vi "Digitizer Fetch and Analyze.vi"(3 "Offset":dbl, 4 "Published Data Id":string[](array[string]), 5 "Vertical Coupling":i32(ring)=1 items=["AC", "DC", "Ground"], 6 "Vertical Range (V)":dbl=2.0 format="%_3g", 7 "Pins":string[](array[string])=["Xout"], 8 "error in (no error)":errorcluster, 9 "Min Record Length":i32=1000 caption="Record Length", 10 "Min. Sample Rate":dbl=1000000.0 caption="Sample Rate" format="%#_6p", 11 "Semiconductor Module Context":T1) -> (0 "error out":errorcluster)   [LabVIEW 2014]
doc: "Example: Measurement Library\n\nRecommended Input Signal: 100 kHz, 2 Vpp, sine wave\n\nDevices Supported: Refer to NI Example Finders\n\nLabVIEW Description:\n\nThis example illustrates fetching scalar measurements from NI-SCOPE, such as period and rise time calculations. \n\nSome common horizontal and vertical parameters are configured for the oscilloscope. The property node is used to set the reference level units, and the low, middle and high reference levels. For more information about measurement library parameters, see the NI-SCOPE VI Reference Help file. \n\nAfter the Read VI is called to acquire a waveform, the Fetch Measurement Stats VI is used to perform the desired scalar measurement analysis on the waveform. NI-SCOPE keeps a history of each measurement's results, which allows it to retrieve the statistics computed over multiple acquisitions. These statistics include the mean, standard deviation, min, max and number of acquisitions used in the statistics. The statistics are updated once per acquisition when the measurement is fetched. The Clear Stats VI clears this history."
uses:
  <vilib>/NI_TestStand_SemiconductorModule/NI_TestStand_Semiconductor_Module.lvlibp/PinMap/General/SemiconductorModuleContext.ctl
  <vilib>/NI_TestStand_SemiconductorModule/NI_TestStand_Semiconductor_Module.lvlibp/PinMap/Advanced/Custom Instruments/GetSessionDataSinglePinSingleInstr.vi
  <instrlib>/niScope/Configure/Trigger/niScope Configure Trigger Immediate.vi
  <instrlib>/niScope/Acquire/niScope Read WDT.vi
  <vilib>/measure/matone.llb/Extract Single Tone Information 1 Chan.vi
  <vilib>/NI_TestStand_SemiconductorModule/NI_TestStand_Semiconductor_Module.lvlibp/PinMap/General/Publish/PublishDataDoubleFunctionalTest.vi
  <vilib>/NI_TestStand_SemiconductorModule/NI_TestStand_Semiconductor_Module.lvlibp
  <vilib>/measure/NI_MAPro.lvlib
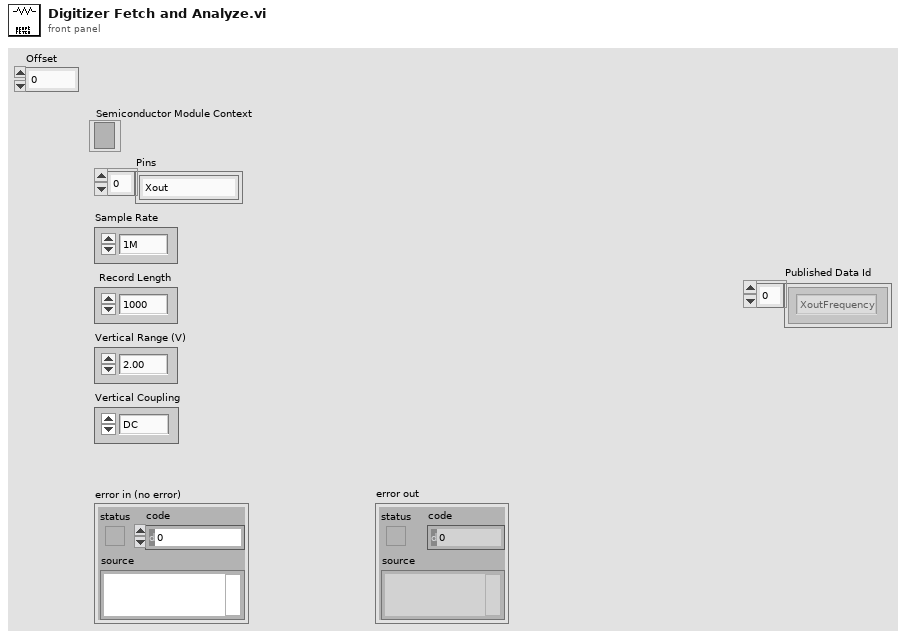
[diagram p1: front panel]
types:
  T1 = typedef "NI_TestStand_Semiconductor_Module.lvlibp/SemiconductorModuleContext.ctl" = refnum<k7>
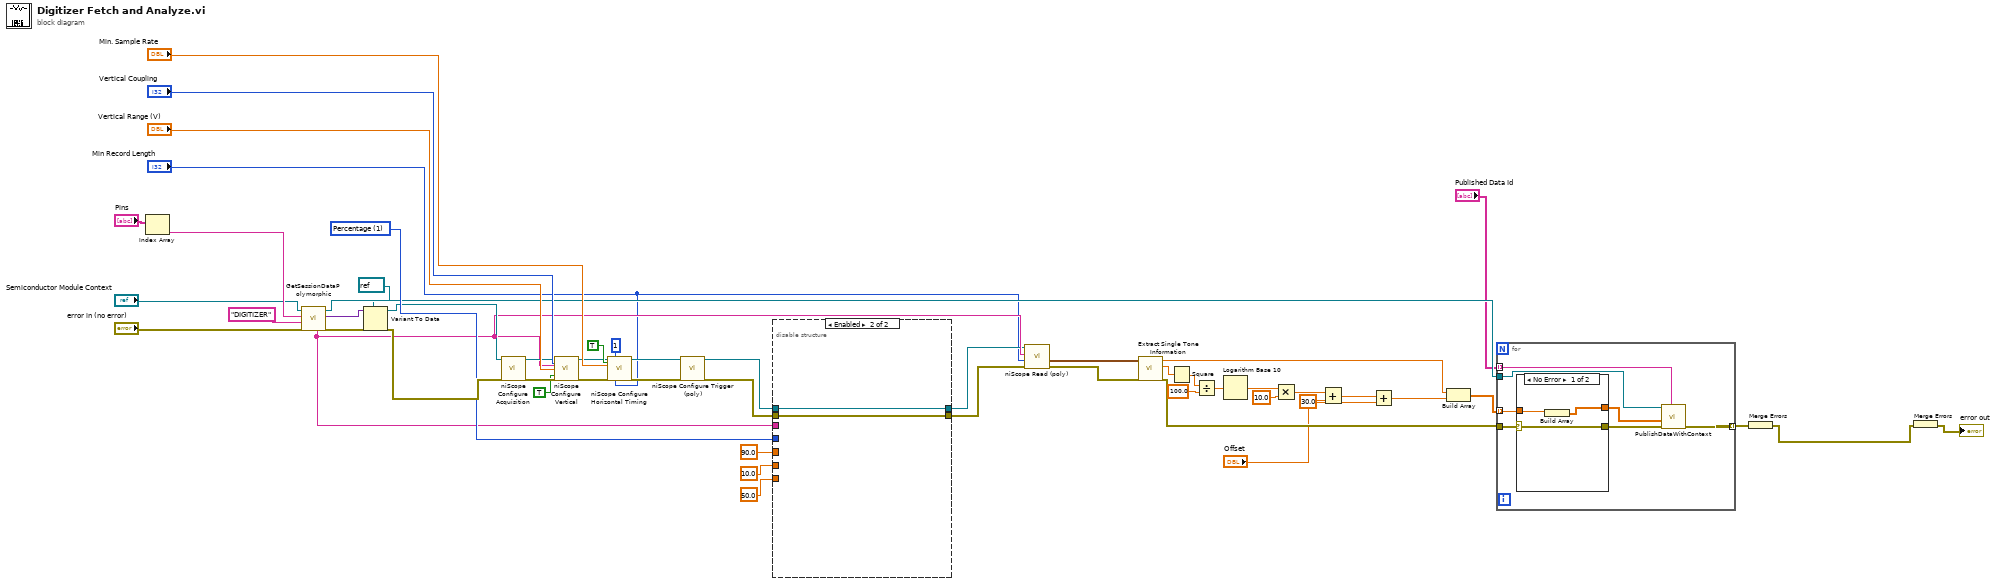
[diagram p0: block diagram]
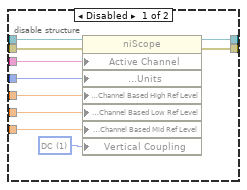
[diagram p2: hidden frame]
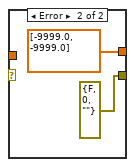
[diagram p3: hidden frame]
diagram:
  w48 = u16 1 items=["Voltage", "Percentage"] ("Reference Level Units")
  n1 = Index Array(array="Pins") -> (element=w38:string)  [unwired: 1 in]
  n2 = call-poly <vilib>:"GetSessionDataPolymorphic.vi"("error in (no error)"="error in (no error)", "Instrument Type Id"="DIGITIZER", "Pin"=w38, "Semiconductor Module Context"="Semiconductor Module Context") -> ("error out"=w52:errorcluster, "Session Data"=w51:variant, "Semiconductor Module Context Out"=w37:T1, "Channel List"=w13:string)  [unwired: 2 in, 2 out]
  n3 = Variant To Data(error in=w52, type=refnum<k15> refnum ("resource name"), Variant=w51) -> (data=w44:refnum<k15>, error out=w53:errorcluster)
  n4 = call <instrlib>:"niScope Configure Acquisition.vi"("instrument handle"=w44, "error in"=w53) -> ("instrument handle out"=w34:refnum<k15>, "error out"=w35:errorcluster)  [unwired: 12 in]
  n5 = call <instrlib>:"niScope Configure Vertical.vi"("instrument handle"=w34, "vertical coupling"="Vertical Coupling", "channels"=w13, "vertical range"="Vertical Range (V)", "error in"=w35, "channel enabled"=TRUE) -> ("instrument handle out"=w21:refnum<k15>, "error out"=w20:errorcluster)  [unwired: 8 in]
  n6 = call <instrlib>:"niScope Configure Horizontal Timing.vi"("instrument handle"=w21, "number of records"=1, "enforce realtime"=TRUE, "min sample rate"="Min. Sample Rate", "error in"=w20, "min record length"="Min Record Length") -> ("instrument handle out"=w33:refnum<k15>, "error out"=w32:errorcluster)  [unwired: 8 in]
  n7 = call-poly <instrlib>:"niScope Configure Trigger (poly).vi"("instrument handle"=w33, "error in"=w32) -> ("instrument handle out"=w10:refnum<k15>, "error out"=w9:errorcluster)  [unwired: 12 in]
  n8 = disable-structure shown="Enabled" {
    disable-tunnel: w48 -> [w63 _]
    disable-tunnel: 90.0 ("High Ref.") -> [w62 _]
    disable-tunnel: 10.0 ("Low Ref.") -> [w61 _]
    disable-tunnel: 50.0 ("Mid Ref.") -> [w60 _]
    disable-tunnel: w13 -> [w58 _]
    disable-tunnel: [w57 w65] -> w11
    disable-tunnel: w10 -> [w56 w65]
    disable-tunnel: w9 -> [w55 w64]
    disable-tunnel: [w54 w64] -> w8
    frame Disabled {
      w59 = 1 items=["AC", "DC", "Ground"] ("Vertical:Vertical Coupling")
      n9 = property class="niScope"(reference=w56, error in=w55, "Active Channel"=w58, "Waveform Measurement:Reference Levels:Units"=w63, "Waveform Measurement:Reference Levels:Channel Based High Ref Level"=w62, "Waveform Measurement:Reference Levels:Channel Based Low Ref Level"=w61, "Waveform Measurement:Reference Levels:Channel Based Mid Ref Level"=w60, "Vertical Coupling"=w59) -> (reference out=w57:refnum<k15>, error out=w54:errorcluster)
    }
    frame Enabled {
    }
  }
  n10 = call-poly <instrlib>:"niScope Read (poly).vi"("error in"=w8, "numSamples"="Min Record Length", "channels"=w13, "instrument handle"=w11) -> ("error out"=w4:errorcluster, "wfm"=w22:waveform(dbl))  [unwired: 4 in, 2 out]
  n11 = call-poly <vilib>:"Extract Single Tone Information.vi"("error in (no error)"=w4, "time signal in"=w22) -> ("error out"=w14:errorcluster, "detected amplitude"=w29:dbl, "detected frequency"=w15:dbl)  [unwired: 4 in, 3 out]
  n12 = Square(x=w29) -> (x^2=w28:dbl)
  n13 = Divide(x=w28, y=100.0) -> (x/y=w26:dbl)
  n14 = Logarithm Base 10(1:w26) -> (0:w25:dbl)
  n15 = Multiply(x=w25, y=10.0) -> (x*y=w23:dbl)
  n16 = Add(x=w23, y=30.0 ("x*y")) -> (x+y=w2:dbl)
  n17 = Add(x=w2, y="Offset") -> (x+y=w3:dbl)
  n18 = Build Array(w15, w3) -> (w17:dbl[])
  n19 = for {
    tunnel: "Published Data Id" -> [w71] mode=indexing
    tunnel: w37 -> [w70]
    tunnel: w17 -> [w69] mode=indexing
    tunnel: w14 -> [w67]
    tunnel: [w72] -> w18 mode=indexing
    n20 = case shown="No Error" w67 {
      selector: w67 -> [w75 _]
      tunnel: [w73 dbl[] [-9999.0, -9999.0]] -> w66
      tunnel: [w75 errorcluster {"status"=FALSE, "code"=0, "source"=""} ("error IO")] -> w68
      tunnel: w69 -> [w74 _]
      frame No Error {
        n21 = Build Array(w74) -> (w73:dbl[])
      }
      frame Error {
      }
    }
    n22 = call-poly <vilib>:"PublishDataWithContext.vi"("Published Data Id"=w71, "error in (no error)"=w68, "Data In"=w66, "Semiconductor Module Context"=w70) -> ("error out"=w72:errorcluster)  [unwired: 6 in, 1 out]
  }
  n23 = Merge Errors(w18) -> (w36:errorcluster)
  n24 = Merge Errors(w36) -> (→"error out":errorcluster)
